vi "test_Bitfile Reload_Scalar Data Type Change.vi"(8 "error in (no error)":errorcluster, 11 "TestCase in":refnum<class "Bitfile Reload System Tests.lvclass">) -> (0 "error out":errorcluster, 3 "TestCase out":refnum<class "Bitfile Reload System Tests.lvclass">)   [LabVIEW 2018, in "Bitfile Reload System Tests.lvclass"]
uses:
  Bitfile Reload System Tests.lvclass
  D:/GitBranches/niveristand-custom-device-testing-tools/VeriStandTestCase/VeriStandTestCase.lvclass
  <vilib>/NI Veristand/Execution/Workspace/NI VeriStand - Get Single Channel Value.vi
  <vilib>/addons/_JKI Toolkits/VI Tester/TestCase.llb/TestCase.lvclass
  FPGA Addon Test Class/FPGA Addon Test Class.lvclass
  <vilib>/NI Veristand/Execution/Workspace/NI_VS Workspace ExecutionAPI.lvlib
  Addon/Addon System Explorer/FPGA Addon System Explorer.lvlib
  C:/Program Files (x86)/National Instruments/LabVIEW 2018/vi.lib/addons/_JKI Toolkits/VI Tester/TestCase.llb/TestCase.lvclass
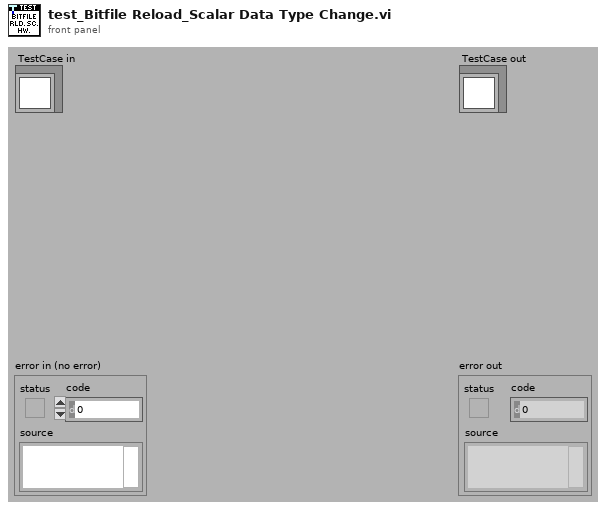
[diagram p1: front panel]
types:
  T1 = typedef "NI_VS Workspace ExecutionAPI.lvlib/WorkspaceAPI.ctl" = refnum<k24>
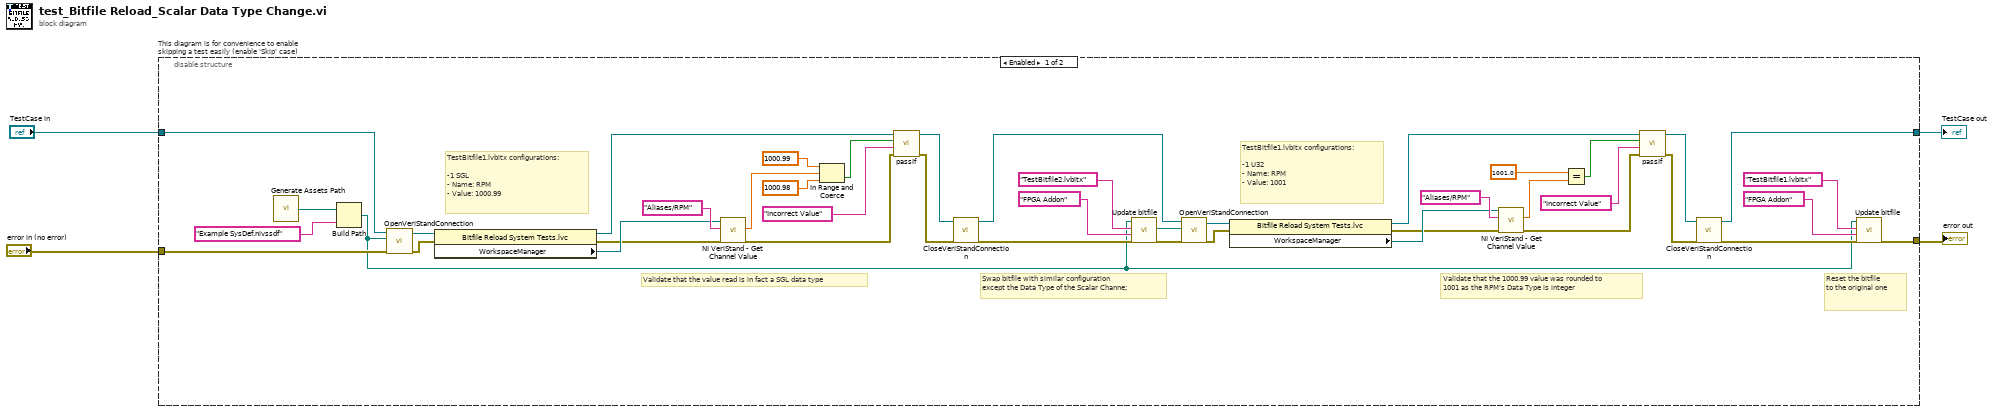
[diagram p0: block diagram]
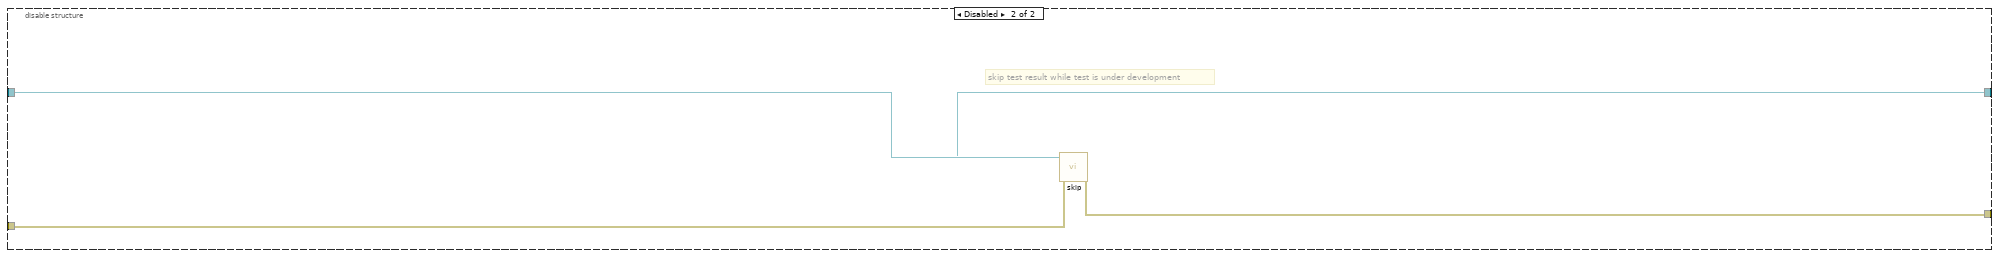
[diagram p2: hidden frame]
diagram:
  n1 = disable-structure "This diagram is for convenience to enable skipping a test easily (enable 'Skip' case)" shown="Enabled" {
    disable-tunnel: "TestCase in" -> [w42 w51]
    disable-tunnel: [w6 w49] -> w1
    disable-tunnel: [w8 w50] -> w3
    disable-tunnel: "error in (no error)" -> [w43 w48]
    frame Enabled {
      # "Reset the bitfile \nto the original one"
      # "Validate that the 1000.99 value was rounded to\n1001 as the RPM's Data Type is integer"
      # "Swap bitfile with similar configuration\nexcept the Data Type of the Scalar Channe;"
      # "Validate that the value read is in fact a SGL data type"
      # "TestBitfile1.lvbitx configurations:\n\n-1 U32\n- Name: RPM\n- Value: 1001"
      # "TestBitfile1.lvbitx configurations:\n\n-1 SGL\n- Name: RPM\n- Value: 1000.99"
      n2 = call "Generate Assets Path.vi"() -> ("Assets path"=w46:path)
      n3 = Build Path(base path=w46, name or relative path="Example SysDef.nivssdf") -> (appended path=w7:path)
      n4 = call-dynamic "OpenVeriStandConnection.vi"("error in (no error)"=w43, "System Definition File"=w7, "VeriStand Test Case in"=w42) -> ("error out"=w30:errorcluster, "VeriStand Test Case out"=w29:refnum<class "Bitfile Reload System Tests.lvclass">)  [unwired: 6 in, 1 out]
      n5 = property class="Bitfile Reload System Tests.lvc"(reference=w29, error in=w30) -> (reference out=w35:refnum<class "Bitfile Reload System Tests.lvclass">, error out=w31:errorcluster, "WorkspaceManager"=w32:T1)
      n6 = call-poly <vilib>:"NI VeriStand - Get Channel Value.vi"("error in (no error)"=w31, "Channel"="Aliases/RPM", "WorkspaceManager in"=w32) -> ("error out"=w34:errorcluster, "Value"=w5:dbl)  [unwired: 6 in, 1 out]
      n7 = In Range and Coerce(upper limit=1000.99, x=w5, lower limit=1000.98) -> (In Range?=w39:bool)  [unwired: 1 out]
      n8 = call-dynamic "passIf.vi"("error in (no error)"=w34, "message (\"\")"="Incorrect Value" ("message (\"\")"), "pass"=w39, "TestCase in"=w35) -> ("error out"=w40:errorcluster, "TestCase out"=w41:refnum<class "Bitfile Reload System Tests.lvclass">)  [unwired: 6 in]
      n9 = call-dynamic "CloseVeriStandConnection.vi"("error in (no error)"=w40, "VeriStand Test Case in"=w41) -> ("error out"=w28:errorcluster, "VeriStand Test Case out"=w17:refnum<class "Bitfile Reload System Tests.lvclass">)  [unwired: 8 in]
      n10 = call "Update bitfile.vi"("error in (no error)"=w28, "FPGA addon name"="FPGA Addon", "bitfile name"="TestBitfile2.lvbitx", "sysdef path in"=w7) -> ("error out"=w13:errorcluster, "sysdef path out"=w12:path)  [unwired: 6 in]
      n11 = call-dynamic "OpenVeriStandConnection.vi"("error in (no error)"=w13, "System Definition File"=w12, "VeriStand Test Case in"=w17) -> ("error out"=w19:errorcluster, "VeriStand Test Case out"=w18:refnum<class "Bitfile Reload System Tests.lvclass">)  [unwired: 6 in, 1 out]
      n12 = property class="Bitfile Reload System Tests.lvc"(reference=w18, error in=w19) -> (reference out=w24:refnum<class "Bitfile Reload System Tests.lvclass">, error out=w20:errorcluster, "WorkspaceManager"=w21:T1)
      n13 = call-poly <vilib>:"NI VeriStand - Get Channel Value.vi"("error in (no error)"=w20, "Channel"="Aliases/RPM", "WorkspaceManager in"=w21) -> ("error out"=w23:errorcluster, "Value"=w16:dbl)  [unwired: 6 in, 1 out]
      n14 = Equal?(x=1001.0, y=w16) -> (x = y?=w14:bool)
      n15 = call-dynamic "passIf.vi"("error in (no error)"=w23, "message (\"\")"="Incorrect Value" ("message (\"\")"), "pass"=w14, "TestCase in"=w24) -> ("error out"=w26:errorcluster, "TestCase out"=w27:refnum<class "Bitfile Reload System Tests.lvclass">)  [unwired: 6 in]
      n16 = call-dynamic "CloseVeriStandConnection.vi"("error in (no error)"=w26, "VeriStand Test Case in"=w27) -> ("error out"=w9:errorcluster, "VeriStand Test Case out"=w6:refnum<class "Bitfile Reload System Tests.lvclass">)  [unwired: 8 in]
      n17 = call "Update bitfile.vi"("error in (no error)"=w9, "FPGA addon name"="FPGA Addon", "bitfile name"="TestBitfile1.lvbitx", "sysdef path in"=w7) -> ("error out"=w8:errorcluster)  [unwired: 6 in, 1 out]
      n18 = call "Reload Bitfile.vi"() -> ()  [unwired: 10 in, 2 out]
    }
    frame Disabled {
      # "skip test result while test is under development"
      n19 = call <vilib>:"skip.vi"("error in (no error)"=w48, "TestCase in"=w51) -> ("error out"=w50:errorcluster, "TestCase out"=w49:refnum<class "Bitfile Reload System Tests.lvclass">)  [unwired: 8 in]
    }
  }
  "error out" <- w3
  "TestCase out" <- w1
